vi "write_session.vi"(8 "error in (no error)":errorcluster caption="entrée d'erreur (pas d'erreur)", 10 "session":refnum<k35>, 11 "Python en entrée":refnum<class "Python.lvclass">) -> (0 "error out":errorcluster caption="sortie d'erreur", 3 "Python en sortie":refnum<class "Python.lvclass">)   [LabVIEW 2020, in "Python.lvclass"]
uses:
  Python.lvclass
  Python.lvclass/Python.ctl
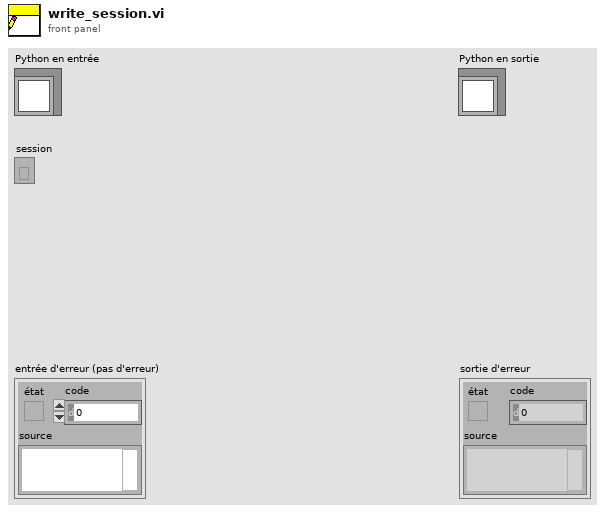
[diagram p1: front panel]
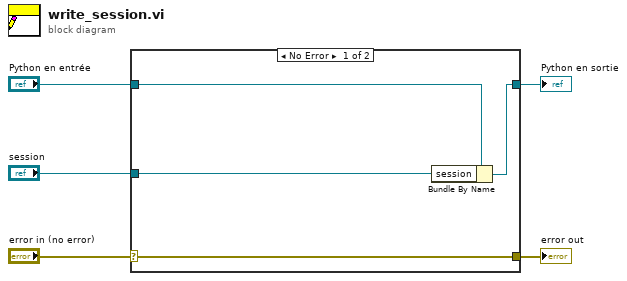
[diagram p0: block diagram]
diagram:
  n1 = case shown="No Error" "error in (no error)" {
    selector: "error in (no error)" -> [w9 w10]
    tunnel: [w9 w10] -> w4
    tunnel: [w7 w11] -> w2
    tunnel: "Python en entrée" -> [w8 w11]
    tunnel: "session" -> [w6 _]
    frame No Error {
      n2 = Bundle By Name(cluster=w8, "session"=w6) -> (w7:refnum<class "Python.lvclass">)
    }
    frame Error {
    }
  }
  "error out" <- w4
  "Python en sortie" <- w2
